vi "SVT Decimated Exp Avg Level.vi"   [LabVIEW 2017]
doc: "Computes the exponential average level of <B>scaled signal [EU]</B> and then decimates the level signal by <B>decimation factor</B>. You can use this polymorphic VI to compute the exponential average level for a single channel or for N channels. The data type you wire to the <B>scaled signal [EU]</B> input determines the polymorphic instance to use."
uses:
  <vilib>/addons/Sound and Vibration/svt_Level/SoundVib_VibrationLevel.lvlib
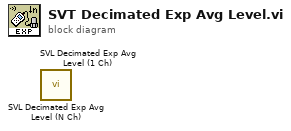
[diagram p0: block diagram]
diagram:
  n1 = call <vilib>:"SVL Decimated Exp Avg Level (N Ch).vi"() -> ()  [unwired: 7 in, 5 out]
  n2 = call <vilib>:"SVL Decimated Exp Avg Level (1 Ch).vi"() -> ()  [unwired: 7 in, 5 out]
